vi "spec_GetData.vi"(8 "error in (no error)":errorcluster, 10 "Detector(s)":string, 11 "instrument in":refnum<class "instrument.lvclass">) -> (0 "error out":errorcluster, 1 "failed?":bool, 2 "value(s)":dbl[](array[numeric]), 3 "instrument out":refnum<class "instrument.lvclass">)   [LabVIEW 2017, in "instrument.lvclass"]
doc: "reads the current value of the detector(s) of the selected spectrometer, returns an array of values.\nIf only one detector was given the array has only one value"
uses:
  instrument.lvclass
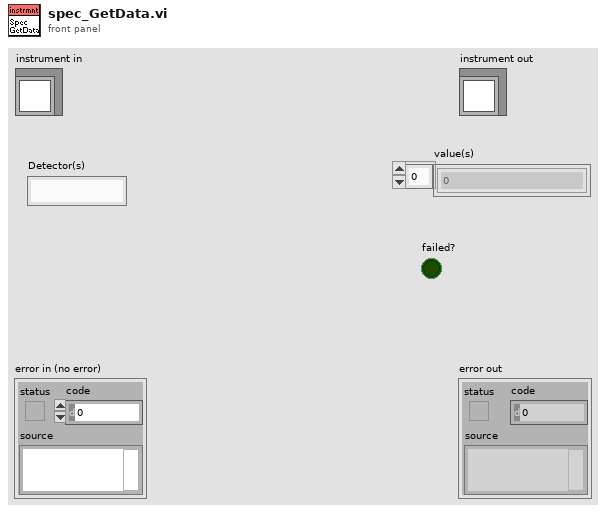
[diagram p1: front panel]
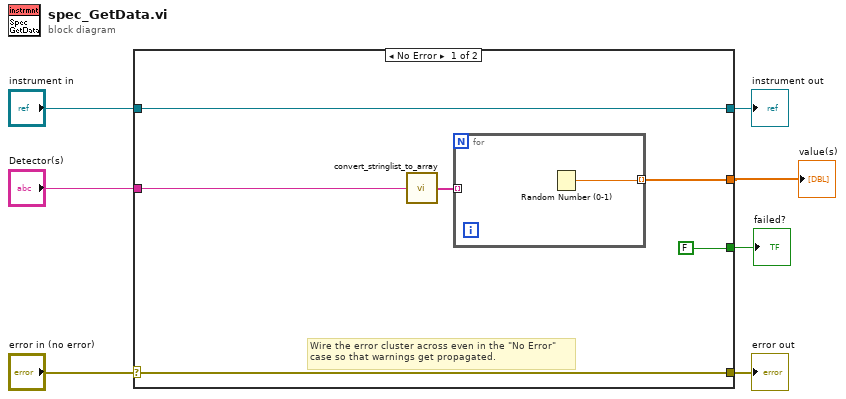
[diagram p0: block diagram]
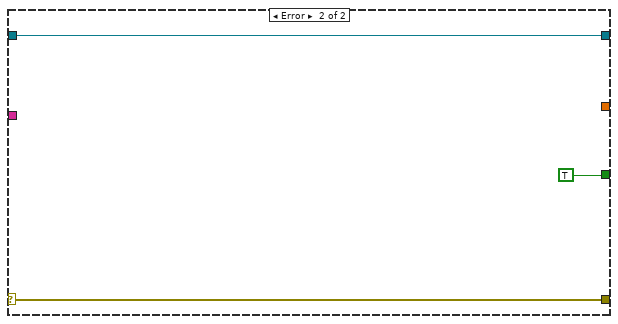
[diagram p2: hidden frame]
diagram:
  n1 = case shown="No Error" "error in (no error)" {
    selector: "error in (no error)" -> [w12 w17]
    tunnel: [w12 w17] -> w6
    tunnel: [w13 w16] -> w4
    tunnel: "instrument in" -> [w13 w16]
    tunnel: [w8 _] -> w1
    tunnel: [FALSE TRUE] -> w3
    tunnel: "Detector(s)" -> [w10 _]
    frame No Error {
      # "Wire the error cluster across even in the \"No Error\"\ncase so that warnings get propagated."
      n2 = call "convert_stringlist_to_array.vi"("string list"=w10) -> ("array of strings"=w9:string[])  [unwired: 4 in]
      n3 = for {
        tunnel: [w14] -> w8 mode=indexing
        tunnel: w9 -> [_] mode=indexing
        n4 = Random Number (0-1)() -> (number: 0 to 1=w14:dbl)
      }
    }
    frame Error {
    }
  }
  "error out" <- w6
  "instrument out" <- w4
  "failed?" <- w3
  "value(s)" <- w1
